vi "Actuator.vi"(11 "to_rio":T1) -> (0 "error out":errorcluster, 1 "time_frame":cluster{"secs":i32, "nsecs":i32}, 2 "set_steering":dbl, 3 "set_speed":dbl, 4 "error 2":i8, 5 "enable":i8, 7 "run":i8)   [LabVIEW 2016]
uses:
  <vilib>/myRIO/Instrument Drivers/Onboard IO/DIO/typedefs/DIO Reference.ctl
  <vilib>/myRIO/Common/Instrument Driver Framework/Utilities/typedefs/myRIO Generic Hardware Reference.ctl
  <vilib>/myRIO/Common/Instrument Driver Framework/Utilities/typedefs/Hardware Version Enum.ctl
  <vilib>/myRIO/Common/Instrument Driver Framework/Utilities/typedefs/myRIO v1.0 Reference.ctl
  <vilib>/myRIO/Common/Instrument Driver Framework/Utilities/typedefs/Generic FPGA Reference.ctl
  <vilib>/myRIO/Common/Instrument Driver Framework/myRIO v1.0/DIO/typedefs/DIO Channels List.ctl
  <vilib>/myRIO/Common/Instrument Driver Framework/myRIO v1.0/DIO/typedefs/DIO Channels Enum.ctl
  <vilib>/userdefined/High Color/nirio_resource_hc.ctl
  <vilib>/myRIO/Instrument Drivers/Onboard IO/PWM/typedefs/PWM Reference.ctl
  <vilib>/myRIO/Common/Instrument Driver Framework/myRIO v1.0/PWM/typedefs/PWM Channels Enum.ctl
  <vilib>/myRIO/Instrument Drivers/Onboard IO/PWM/typedefs/PWM Configuration.ctl
  <vilib>/myRIO/Common/Instrument Driver Framework/Utilities/vis/Is FPGA Ref Available.vi
  <vilib>/myRIO/Common/Instrument Driver Framework/roboRIO v1.0/DIO/vis/roboRIO v1.0 Open DIO.vi
  <vilib>/myRIO/Instrument Drivers/Onboard IO/DIO/vis/Write.vi
  <vilib>/myRIO/Common/Instrument Driver Framework/roboRIO v1.0/PWM/vis/roboRIO v1.0 Open PWM.vi
  <vilib>/myRIO/Instrument Drivers/Onboard IO/PWM/vis/Set Duty Cycle and Frequency.vi
  <vilib>/myRIO/Common/Instrument Driver Framework/Utilities/vis/Validate Channels.vi
  <vilib>/myRIO/Common/Instrument Driver Framework/roboRIO v1.0/DIO/vis/roboRIO v1.0 Reserve DIO.vi
  <vilib>/myRIO/Common/Instrument Driver Framework/roboRIO v1.0/PWM/vis/roboRIO v1.0 Reserve PWM.vi
  <vilib>/myRIO/Common/Instrument Driver Framework/roboRIO v1.0/DIO/vis/roboRIO v1.0 Build MUX Configuration DIO.vi
  <vilib>/myRIO/Common/Instrument Driver Framework/roboRIO v1.0/Resource Manager/vis/roboRIO v1.0 Reserve Channel List.vi
  <vilib>/myRIO/Common/Instrument Driver Framework/roboRIO v1.0/PWM/vis/roboRIO v1.0 Build MUX Configuration PWM.vi
  <vilib>/myRIO/Common/Instrument Driver Framework/roboRIO v1.0/Resource Manager/vis/roboRIO v1.0 Create Configuration List.vi
  <vilib>/myRIO/Common/Instrument Driver Framework/roboRIO v1.0/Resource Manager/vis/roboRIO v1.0 Reserve Channel.vi
  <vilib>/myRIO/Common/Instrument Driver Framework/roboRIO v1.0/Resource Manager/vis/roboRIO v1.0 Unreserve Channel.vi
  <vilib>/myRIO/Common/Instrument Driver Framework/roboRIO v1.0/Resource Manager/vis/roboRIO v1.0 Build Mutex Name.vi
  <vilib>/Utility/VariantDataType/GetNumericInfo.vi
  <vilib>/Utility/error.llb/Error Cluster From Error Code.vi
  <vilib>/myRIO/Common/Instrument Driver Framework/roboRIO v1.0/roboRIO v1.0 Open.vi
  <vilib>/myRIO/Common/Instrument Driver Framework/Utilities/vis/IO Manager.vi
  <vilib>/myRIO/Common/Instrument Driver Framework/Utilities/vis/Configuration Manager.vi
  <vilib>/myRIO/Common/Instrument Driver Framework/roboRIO v1.0/Resource Manager/vis/roboRIO v1.0 Configure IO.vi
  <vilib>/myRIO/Common/Instrument Driver Framework/myRIO v1.0/myRIO v1.0 Close.vi
  <vilib>/myRIO/Common/Instrument Driver Framework/roboRIO v1.0/PWM/vis/roboRIO v1.0 Write PWM.vi
  <vilib>/myRIO/Common/Instrument Driver Framework/roboRIO v1.0/DIO/vis/roboRIO v1.0 Write DIO.vi
  <vilib>/myRIO/Express VI/Onboard IO/PWM/PWM Express VI.xnode
  <vilib>/myRIO/Instrument Drivers/Onboard IO/PWM/vis/myRIO PWM Open.xnode
  <vilib>/myRIO/Express VI/Onboard Devices/LED/LED Express VI.xnode
  <vilib>/myRIO/Instrument Drivers/Onboard IO/DIO/vis/myRIO DIO Open.xnode
  <vilib>/myRIO/Instrument Drivers/Onboard IO/PWM/PWM.lvlib
  <vilib>/myRIO/Instrument Drivers/Onboard IO/DIO/DIO.lvlib
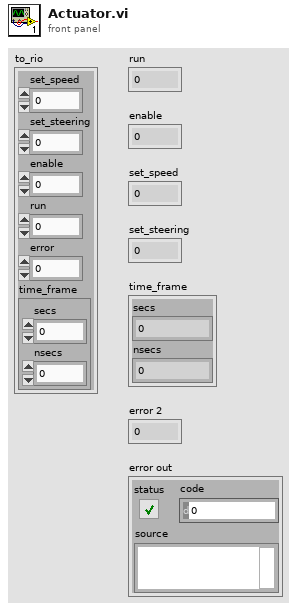
[diagram p1: front panel]
types:
  T1 = cluster{"set_speed":dbl, "set_steering":dbl, "enable":i8, "run":i8, "error":i8, "time_frame":cluster{"secs":i32, "nsecs":i32}}
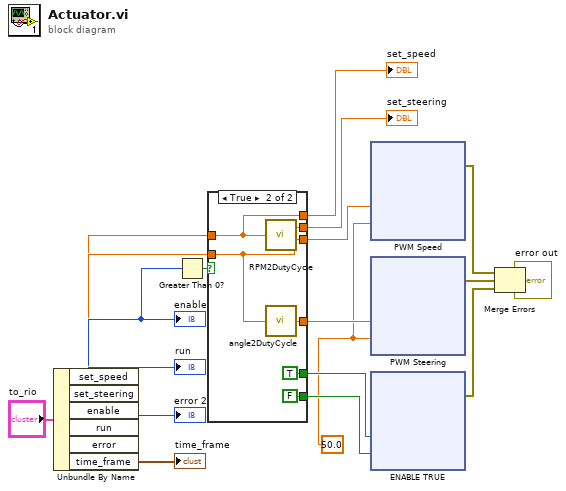
[diagram p0: block diagram]
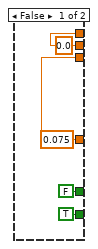
[diagram p2: hidden frame]
diagram:
  w1 = 50.0 ("Frequency [Hz]")
  n1 = Unbundle By Name("to_rio") -> ("set_speed"=w15:dbl, "set_steering"=w16:dbl, "enable"=w17:i8, "run"=→"run":i8, "error"=→"error 2":i8, "time_frame"=→"time_frame":cluster{"secs":i32, "nsecs":i32})
  "enable" <- w17
  n2 = Greater Than 0?(x=w17) -> (x > 0?=w9:bool)
  n3 = case shown="True" w9 {
    tunnel: [w23 w29] -> w5
    tunnel: [w23 w28] -> w6
    tunnel: [w22 w24] -> w7
    tunnel: [w22 w25] -> w8
    tunnel: [FALSE ("RADIO (Green)") TRUE ("RADIO (Green)")] -> w10
    tunnel: [TRUE ("RADIO (Red)") FALSE ("RADIO (Red)")] -> w11
    tunnel: w15 -> [_ w25]
    tunnel: w16 -> [_ w24]
    frame False {
      w22 = 0.0
      w23 = 0.075
    }
    frame True {
      n4 = call "RPM2DutyCycle.vi"("Speed"=w25) -> ("Duty Cycle"=w28:dbl)
      n5 = call "angle2DutyCycle.vi"("Steering Angle"=w24) -> ("Duty Cycle"=w29:dbl)
    }
  }
  "set_speed" <- w8
  "set_steering" <- w7
  n6 = xnode "PWM Speed"("Duty Cycle"=w6, "Frequency [Hz]"=w1) -> ("error out"=w2:errorcluster)  [unwired: 1 in]
  n7 = xnode "PWM Steering"("Duty Cycle"=w5, "Frequency [Hz]"=w1) -> ("error out"=w3:errorcluster)  [unwired: 1 in]
  n8 = xnode "ENABLE TRUE"("RADIO (Green)"=w10, "RADIO (Red)"=w11) -> ("error out"=w12:errorcluster)  [unwired: 1 in]
  n9 = Merge Errors(w2, w3, w12) -> (→"error out":errorcluster)
